vi "histogram and threshold grab.vi"() -> ()   [LabVIEW 2013]
uses:
  <vilib>/vision/NI_Vision_Development_Module.lvlib
panel:
  in  "Range (Threshold 1)":cluster{"Lower value":sgl, "Upper value":sgl}={"Lower value"=0.0, "Upper value"=128.0}
  out "histogram":T1(graph)
  out "ms between image":u32
  out "Frame Rate":dbl
  in  "Stop (F)":bool
  out "Image Out":T2(plugin-control)
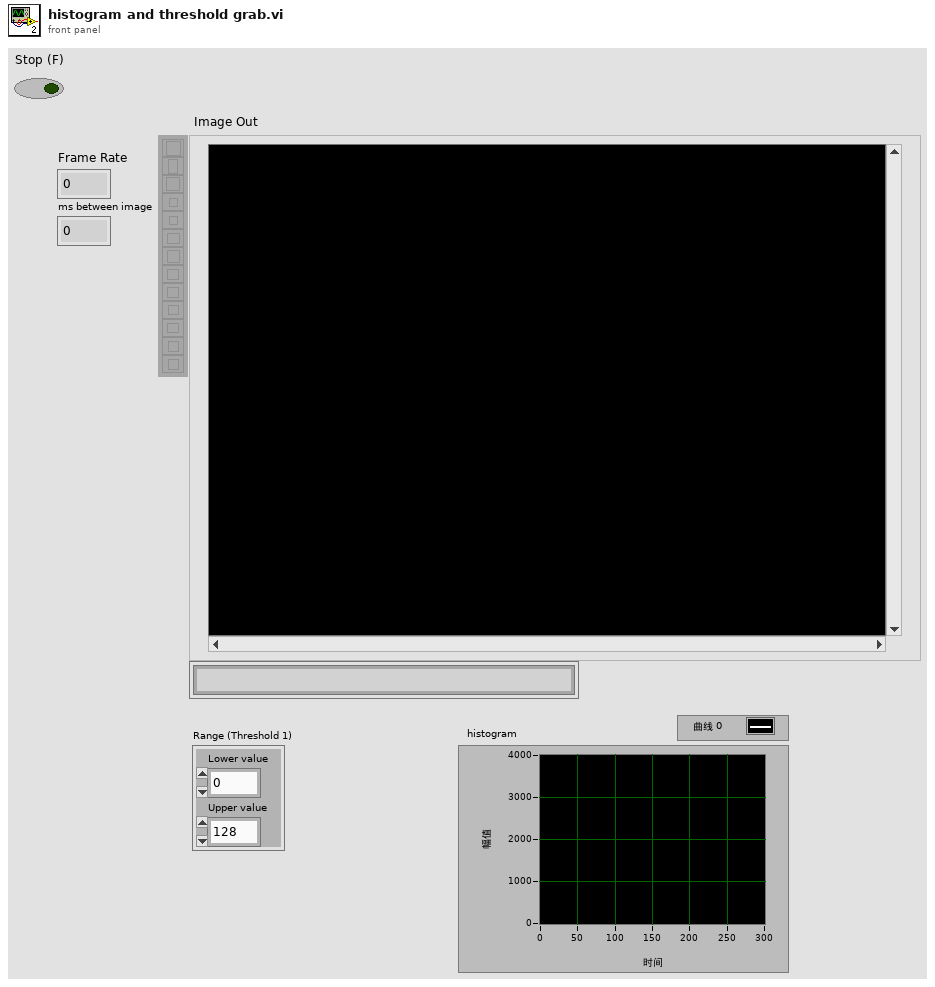
[diagram p1: front panel]
types:
  T1 = cluster{"Starting Value":sgl, "Incremental Value":sgl, "Histogram":u32[]}
  T2 = typedef "IMAQ Image.ctl" = refnum<image>
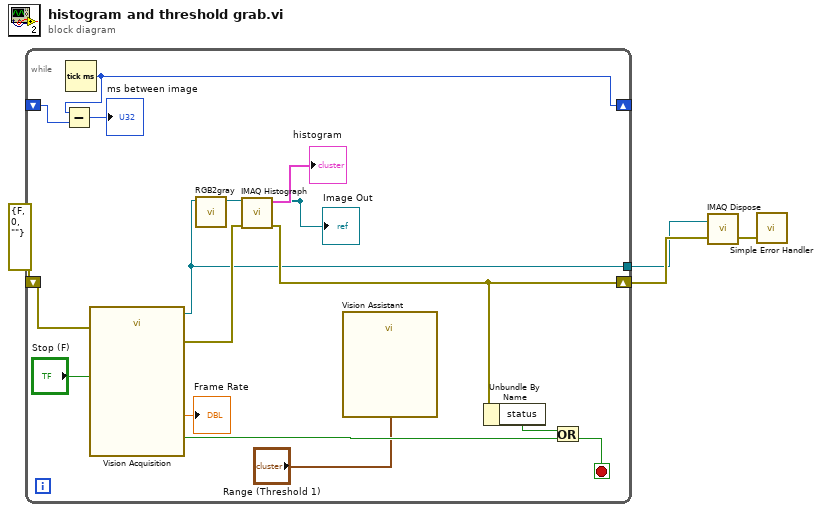
[diagram p0: block diagram]
diagram:
  n1 = while {
    shift-right: [w16] -> _
    shift-left: _ -> [w15]
    shift-right: [w9] -> w4
    shift-left: errorcluster {"status"=FALSE, "code"=0, "source"=""} ("error out") -> [w12]
    tunnel: [w7] -> w2
    stop <- w13 stop-if-true
    n2 = Tick Count (ms)() -> (millisecond timer value=w16:u32)
    n3 = Subtract(x=w16, y=w15) -> (x-y=→"ms between image":u32)
    n4 = call "Vision Acquisition"("Stop (F)"="Stop (F)", "error in"=w12) -> ("Image Out"=w7:T2, "Frame Rate"=→"Frame Rate":dbl, "Stopped"=w18:bool, "error out"=w10:errorcluster)  [unwired: 22 in]
    n5 = call "RGB2gray.vi"("引用句柄输入"=w7) -> ("引用句柄输出"=w6:T2)  [unwired: 10 in]
    "Image Out" <- w6
    n6 = call "IMAQ Histograph"("error in (no error)"=w10, "Image"=w6) -> ("error out"=w9:errorcluster, "Histogram Graph"=→"histogram":T1)  [unwired: 6 in, 2 out]
    n7 = call "Vision Assistant"("Range (Threshold 1)"="Range (Threshold 1)") -> ()  [unwired: 25 in, 2 out]
    n8 = Unbundle By Name(w9) -> ("status"=w11:bool)
    n9 = Or(x=w11, y=w18) -> (x .or. y?=w13:bool)
  }
  n10 = call "IMAQ Dispose"("Image"=w2, "error in (no error)"=w4) -> ("error out"=w1:errorcluster)  [unwired: 4 in]
  n11 = call <vilib>:"Simple Error Handler.vi"("error in (no error)"=w1) -> ()  [unwired: 4 in, 5 out]
